vi "ProcesMTData9_2.vi"() -> ()   [LabVIEW 2018]
uses:
  <vilib>/gmath/NumericalOptimization/Nonlinear Curve Fit LM.vi
  <vilib>/gmath/statdist.llb/st_Percentiles (scalar).vi
  <vilib>/gmath/NI_Gmath.lvlib
panel:
  out "Busy with":string
  in  "test":bool
  out "Busy":bool
  in  "Fit function":u16(ring) caption="Data set" items=["Choose model ...", "WLC", "FiberWLC"]
  out "Parametersclipboard":T1(array[cluster])
  in  "Parameters":T1(array[cluster]) {"value" format="%#.2f"; "SE" format="%_2g"}
  out "Cursor positions label":string[](array[string])=["t min (s)", "t max (s)", "F min (pN)", "Fmax (pN)", "z min (um)", "z max (um)"]
  in  "Cursor positions":dbl[](array[numeric])=[0.0, 200.0, 0.0, 25.0, 0.0, 2.0]
  in  "Data set":u16(ring) caption="Trace name"
  out "F(z) graph":cluster{"Data Out":dbl[], "Data Out":dbl[]}[](graph) caption="<65535>\n\nChoose model ..."
  out "z(t) Graph":cluster{"Data Out":dbl[], "Data Out":dbl[]}[](graph)
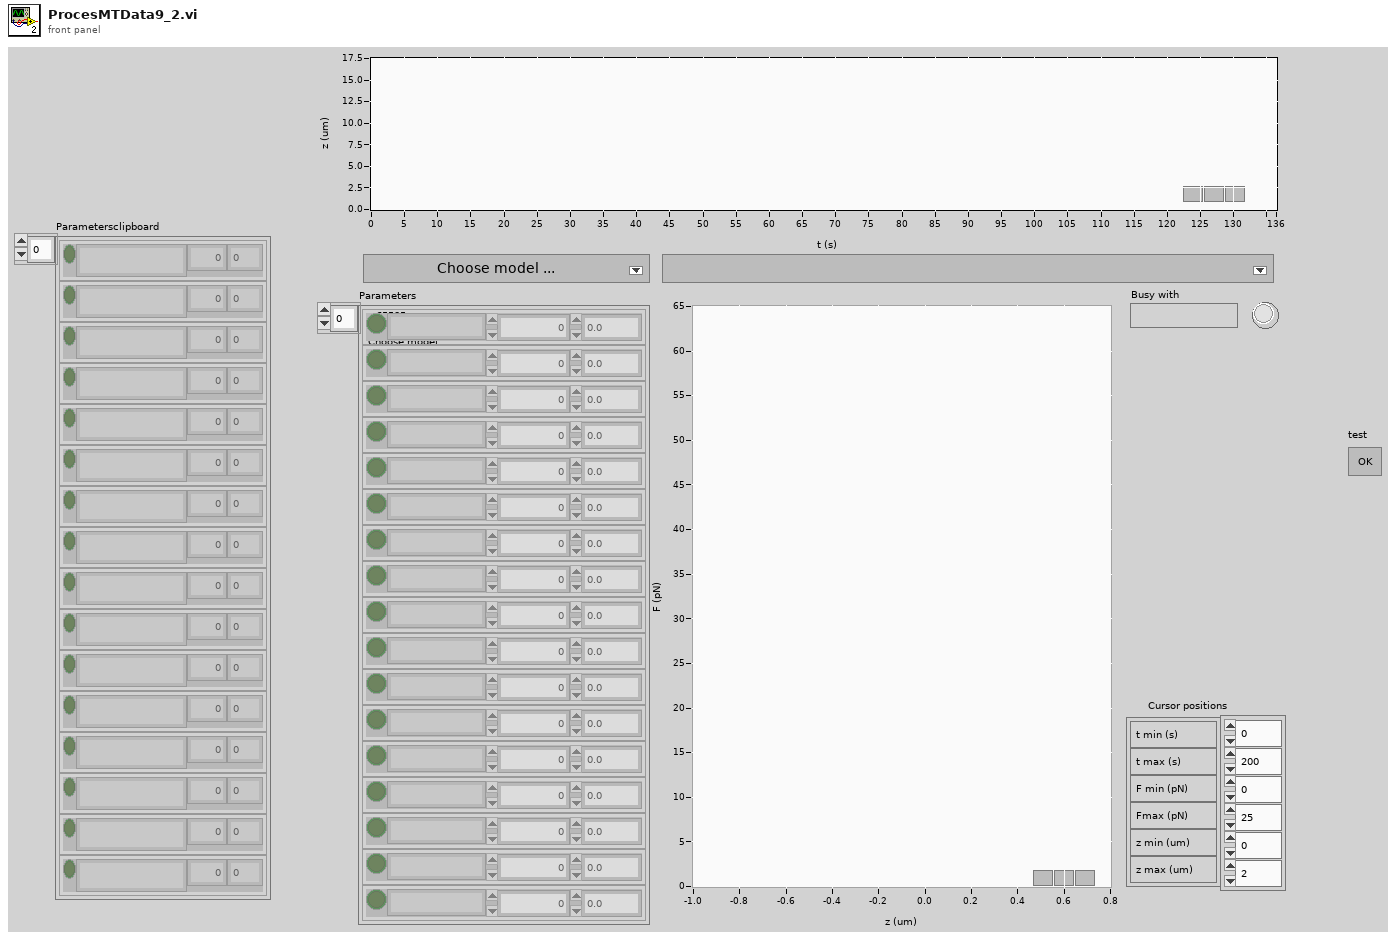
[diagram p1: front panel]
types:
  T1 = cluster{"fit":bool, "parname":string, "value":dbl, "SE":dbl}[]
  T2 = enum16{"Select all", "Select none", "Include", "Exclude"}
  T3 = enum16{"Init", "Reset", "Update var pars", "Update SE's", "Get", "Save to file", "Read from file"}
  T4 = enum16{"Read", "Write", "Get channels", "Delete channels"}
  T5 = cluster{"fit":bool, "parname":string, "value":dbl, "SE":dbl}
  T6 = cluster{bool, "ParName":string, "Value":dbl, "SE":dbl}[]
  T7 = typedef "eventvkey.ctl" = enum16{"ASCII", "Enter", "Return", "Shift", "Ctrl", "Alt", "Cmd", "Opt", "Caps", "NumLock", "Clear", "Break", "Up", "Down", "Left", "Right", "Insert", "Delete", "Home", "End", "PageUp", "PageDown", "Escape", "Help", "Pause", "ScrollLock", "F1", "F2", "F3", "F4", "F5", "F6", "F7", "F8", "F9", "F10", "F11", "F12", "F13", "F14", "F15", "F16", "F17", "F18", "F19", "F20", "F21", "F22", "F23", "F24", "Play", "VolumeUp", "VolumeDown", "Mute", "Two Byte Char"}
  T8 = enum16{"Init", "Update", "Get", "Save", "Add SE", "To text"}
  T9 = enum16{"Init", "Update", "Get", "Save", "Add SE"}
  T10 = typedef "NI_Matrix.lvlib/RealMatrix.ctl" = dbl[][]
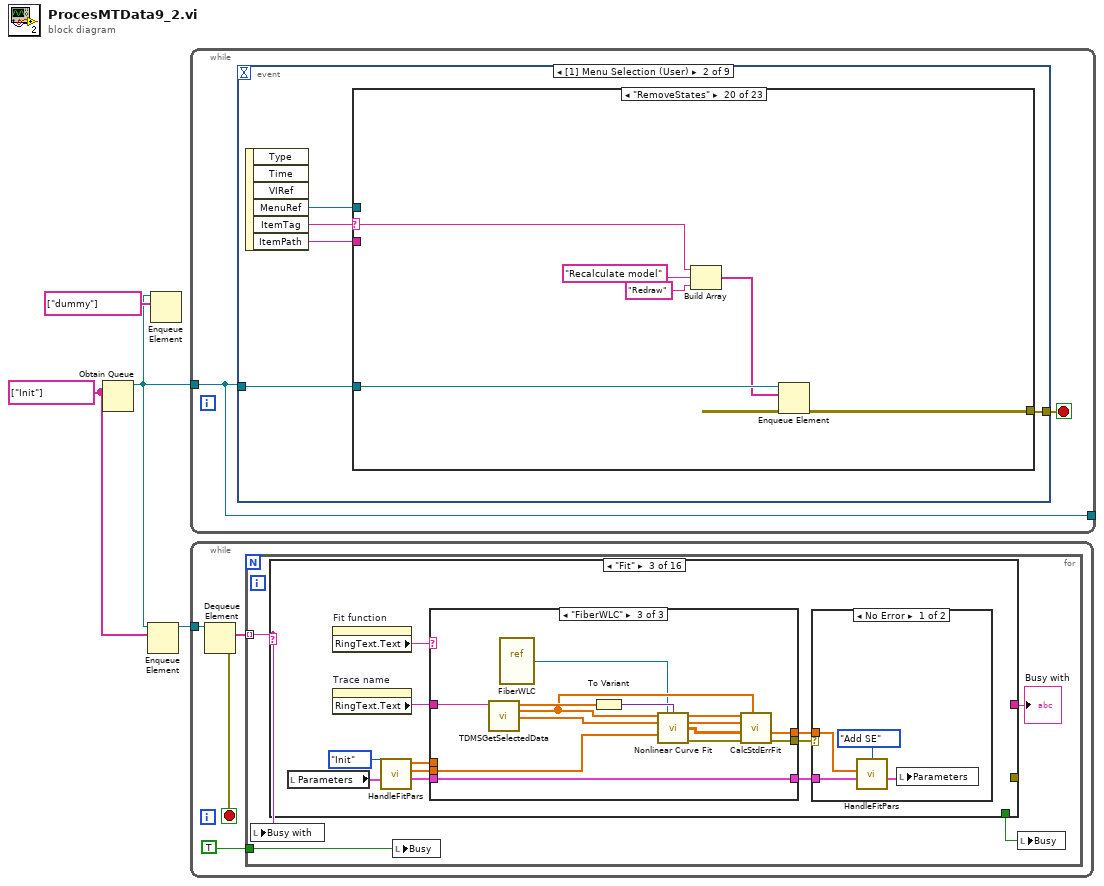
[diagram p0: block diagram]
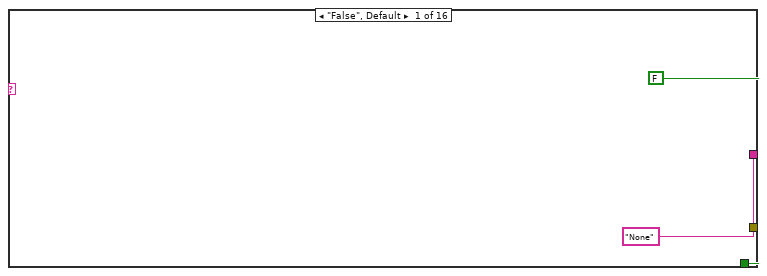
[diagram p2: hidden frame]
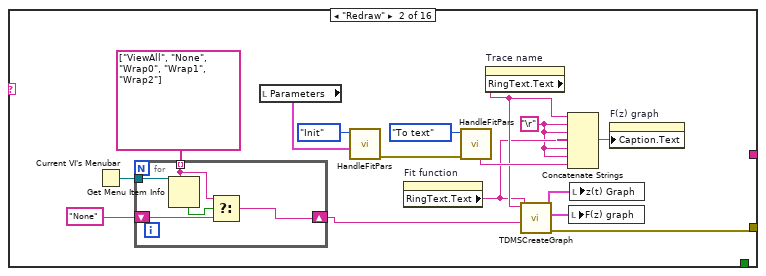
[diagram p3: hidden frame]
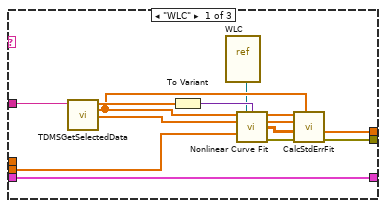
[diagram p4: hidden frame]
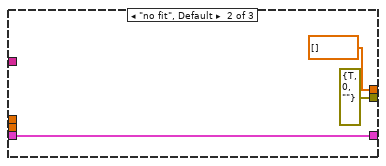
[diagram p5: hidden frame]
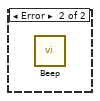
[diagram p6: hidden frame]
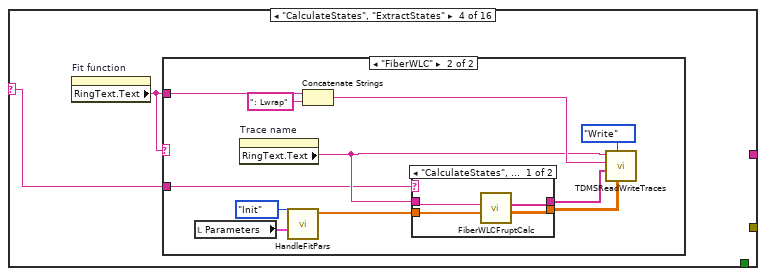
[diagram p7: hidden frame]
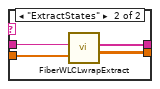
[diagram p9: hidden frame]
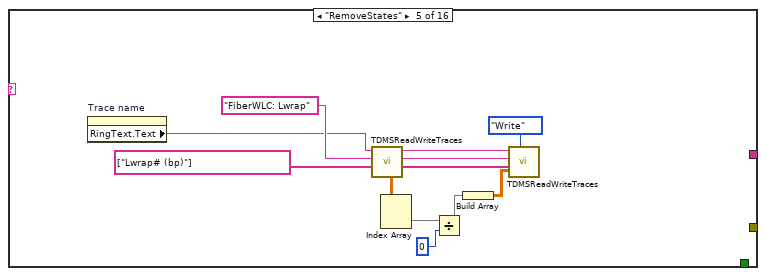
[diagram p10: hidden frame]
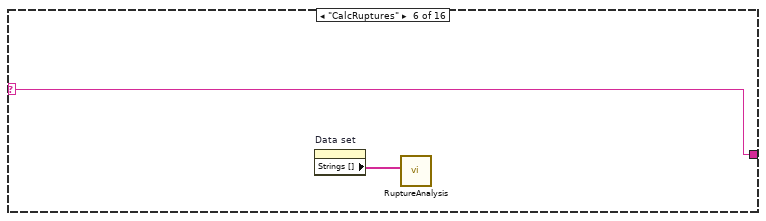
[diagram p11: hidden frame]
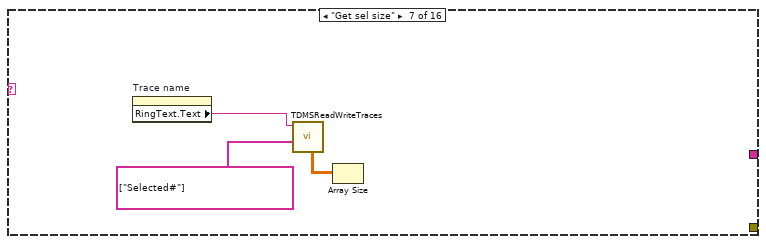
[diagram p12: hidden frame]
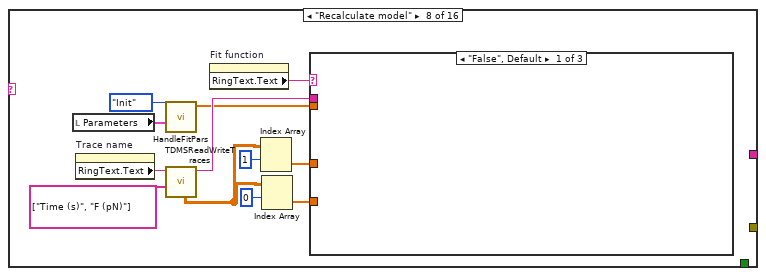
[diagram p13: hidden frame]
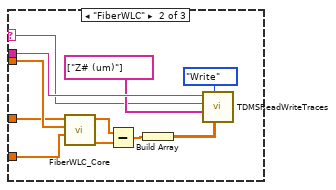
[diagram p14: hidden frame]
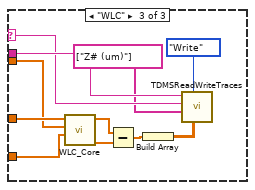
[diagram p15: hidden frame]
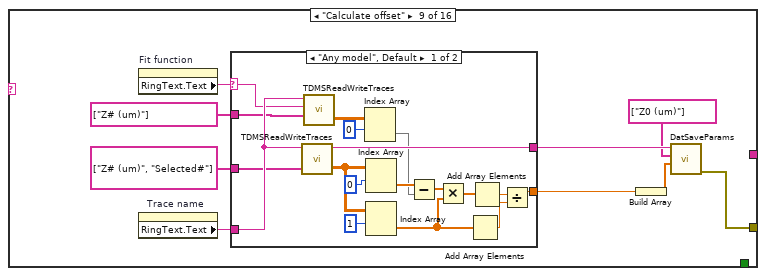
[diagram p16: hidden frame]
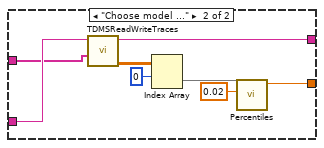
[diagram p17: hidden frame]
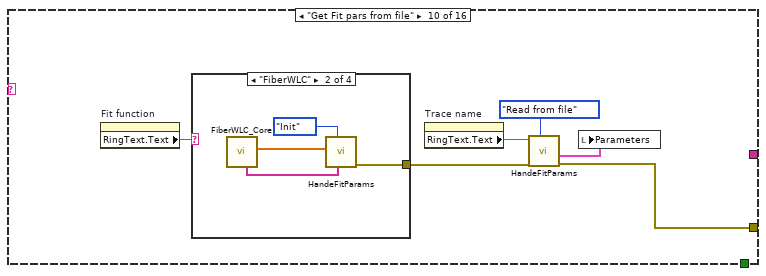
[diagram p18: hidden frame]
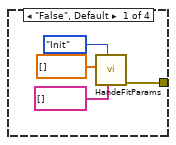
[diagram p19: hidden frame]
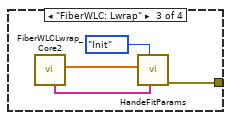
[diagram p20: hidden frame]
diagram:
  w3 = string[] ["Init"]
  n1 = Obtain Queue(element data type=w3) -> (queue out=w1:refnum<queue>)  [unwired: 4 in, 2 out]
  n2 = Enqueue Element(queue=w1, element=w3) -> (queue out=w4:refnum<queue>)  [unwired: 2 in, 2 out]
  n3 = Enqueue Element(queue=w1, element=string[] ["dummy"]) -> ()  [unwired: 2 in, 3 out]
  n4 = while {
    tunnel: w1 -> [w5]
    tunnel: [w5] -> _
    stop <- w6 stop-if-true
    n5 = event shown="[1] Menu Selection (User)" {
      selector: _ -> [_ _ _ _ _ _ _ _ _]
      dyn-events: _ -> [_ _ _ _ _ _ _ _ _]
      timeout: _ -> [_ _ _ _ _ _ _ _ _]
      tunnel: [_ w9 _ _ w399 w405 w429 _ w460] -> w6
      tunnel: w5 -> [_ w7 w376 _ w400 w407 w431 w439 w461]
      event Timeout {
        n6 = event-data() -> ()  [unwired: 1 in, 2 out]
      }
      event Menu Selection (User) {
        n7 = event-data() -> ("MenuRef"=w10:refnum<k9>, "ItemTag"=w11:string, "ItemPath"=w8:string)  [unwired: 1 in, 3 out]
        n8 = case shown="\"RemoveStates\"" w11 {
          selector: w11 -> [w17 w147 _ _ _ w180 _ _ _ _ _ _ _ _ w235 _ _ _ w307 w314 w320 w363 _]
          tunnel: w10 -> [_ w151 _ _ _ _ _ _ _ _ _ _ _ _ _ _ _ _ _ _ _ w364 _]
          tunnel: [_ _ _ _ _ _ _ _ _ _ _ errorcluster {"status"=TRUE, "code"=0, "source"=""} ("error out") _ w228 w236 w248 _ w304 w309 w315 _ _ _] -> w9
          tunnel: w8 -> [_ _ _ _ _ _ _ _ _ _ _ _ _ _ _ _ _ _ _ _ _ _ _]
          tunnel: w7 -> [w15 w145 w161 w171 w173 w176 _ _ w209 w211 _ w218 _ _ _ w250 _ w305 w310 w316 _ _ _]
          frame "Add", "All", "Constant", "Current view", "Decreasing", "Exclude", "Include", "Increasing", "Invert", "Subtract" {
            n9 = local read "Cursor positions"() -> (w16:dbl[])
            n10 = property on="Trace name" class="Ring (strict)"() -> ("RingText.Text"=w12:string)  [unwired: 2 in, 2 out]
            n11 = case shown="\"Decreasing\"" w17 {
              tunnel: w16 -> [w21 w25 w29 w38 w72 _ _ _ _ w142]
              tunnel: w12 -> [w20 w24 w28 w35 w73 w85 w99 w114 w128 w143]
              tunnel: [w18 w22 w26 w30 w62 w77 w90 w104 w119 w132] -> w13
              frame "Include", Default {
                n12 = call "TDMSSetSelection.vi"("task"=T2."Include", "min/max [t, F, z]"=w21, "tracename in"=w20) -> ("error out"=w18:errorcluster)  [unwired: 6 in, 2 out]
              }
              frame "All" {
                n13 = call "TDMSSetSelection.vi"("task"=T2."Select all", "min/max [t, F, z]"=w25, "tracename in"=w24) -> ("error out"=w22:errorcluster)  [unwired: 6 in, 2 out]
              }
              frame "Exclude" {
                n14 = call "TDMSSetSelection.vi"("task"=T2."Exclude", "min/max [t, F, z]"=w29, "tracename in"=w28) -> ("error out"=w26:errorcluster)  [unwired: 6 in, 2 out]
              }
              frame "Current view" {
                n15 = property on="F(z) graph" class="XYGraph (strict)"() -> ("YScale.Minimum"=w40:dbl, "YScale.Maximum"=w39:dbl, "XScale.Minimum"=w33:dbl, "XScale.Maximum"=w32:dbl)  [unwired: 2 in, 2 out]
                n16 = property on="z(t) Graph" class="XYGraph (strict)"() -> ("XScale.Minimum"=w42:dbl, "XScale.Maximum"=w41:dbl)  [unwired: 2 in, 2 out]
                n17 = Build Array(w42, w41, w40, w39, w33, w32) -> (w36:dbl[])
                n18 = Replace Array Subset(array=w38, new element=w36, index=0) -> (w34:dbl[])
                n19 = local write "Cursor positions"(w34) -> ()
                n20 = for {
                  tunnel: w34 -> [w43] mode=indexing
                  i -> [w44]
                  n21 = case shown="4, 5" w44 {
                    selector: w44 -> [w46 w52 w57]
                    tunnel: w43 -> [w45 w48 w53]
                    frame 0, Default {
                      n22 = property on="z(t) Graph" class="XYGraph (strict)"("Active Cursor"=w46) -> (error out=w47:errorcluster)  [unwired: 2 in, 1 out]
                      n23 = property on="z(t) Graph" class="XYGraph (strict)"(error in=w47, "Cursor.Cursor X"=w45) -> ()  [unwired: 1 in, 2 out]
                    }
                    frame 2, 3 {
                      n24 = Subtract(x=w52, y=2) -> (x-y=w49:i32)
                      n25 = property on="F(z) graph" class="XYGraph (strict)"("Active Cursor"=w49) -> (error out=w50:errorcluster)  [unwired: 2 in, 1 out]
                      n26 = property on="F(z) graph" class="XYGraph (strict)"(error in=w50, "Cursor.Cursor Y"=w48) -> ()  [unwired: 1 in, 2 out]
                    }
                    frame 4, 5 {
                      n27 = Subtract(x=w57, y=4) -> (x-y=w54:i32)
                      n28 = property on="F(z) graph" class="XYGraph (strict)"("Active Cursor"=w54) -> (error out=w55:errorcluster)  [unwired: 2 in, 1 out]
                      n29 = property on="F(z) graph" class="XYGraph (strict)"(error in=w55, "Cursor.Cursor X"=w53) -> ()  [unwired: 1 in, 2 out]
                    }
                  }
                }
                n30 = call "TDMSSetSelection.vi"("task"=T2."Include", "min/max [t, F, z]"=w34, "tracename in"=w35) -> ("error out"=w30:errorcluster)  [unwired: 6 in, 2 out]
              }
              frame "Subtract" {
                w61 = string[] ["Selected#"]
                n31 = call "TDMSReadWriteTraces.vi"("Channels in"=w61, "tracename"=w73) -> ("tracename out"=w64:string, "Data out"=w71:dbl[][])  [unwired: 4 in, 4 out]
                n32 = call "TDMSSetSelection.vi"("task"=T2."Include", "min/max [t, F, z]"=w72, "tracename in"=w64) -> ("Selected"=w69:dbl[])  [unwired: 6 in, 2 out]
                n33 = Index Array(array=w71) -> (element=w68:dbl[])  [unwired: 2 in]
                n34 = Subtract(x=w68, y=w69) -> (x-y=w67:dbl[])
                n35 = Equal?(x=1.0, y=w67) -> (x = y?=w65:bool[])
                n36 = Boolean To (0,1)(Boolean=w65) -> (0, 1=w60:i16[])
                n37 = Build Array(w60) -> (w59:i16[][])
                n38 = call "TDMSReadWriteTraces.vi"("Data in"=w59, "Task"=enum16{"Read", "Write"}."Write", "Channels in"=w61, "group name"="Selections", "tracename"=w64) -> ("error out"=w62:errorcluster)  [unwired: 1 in, 5 out]
              }
              frame "Invert" {
                w76 = string[] ["Selected#"]
                n39 = call "TDMSReadWriteTraces.vi"("Channels in"=w76, "tracename"=w85) -> ("tracename out"=w84:string, "Data out"=w79:dbl[][])  [unwired: 4 in, 4 out]
                n40 = Index Array(array=w79, index (row)=0) -> (element=w78:dbl[])  [unwired: 1 in]
                n41 = Equal To 0?(x=w78) -> (x = 0?=w83:bool[])
                n42 = Boolean To (0,1)(Boolean=w83) -> (0, 1=w82:i16[])
                n43 = Build Array(w82) -> (w75:i16[][])
                n44 = call "TDMSReadWriteTraces.vi"("Data in"=w75, "Task"=enum16{"Read", "Write"}."Write", "Channels in"=w76, "group name"="Selections", "tracename"=w84) -> ("error out"=w77:errorcluster)  [unwired: 1 in, 5 out]
              }
              frame "Decreasing" {
                n45 = call "TDMSReadWriteTraces.vi"("Channels in"=string[] ["F (pN)"], "tracename"=w99) -> ("tracename out"=w97:string, "Data out"=w98:dbl[][])  [unwired: 4 in, 4 out]
                n46 = Index Array(array=w98) -> (element=w95:dbl[])  [unwired: 2 in]
                n47 = call "Getdxdtd2dt2.vi"("Data in"=w95) -> ("first derivative"=w94:dbl[])  [unwired: 3 in, 1 out]
                n48 = Less?(x=w94, y=0.0) -> (x < y?=w93:bool[])
                n49 = Boolean To (0,1)(Boolean=w93) -> (0, 1=w92:i16[])
                n50 = Build Array(w92) -> (w88:i16[][])
                n51 = call "TDMSReadWriteTraces.vi"("Data in"=w88, "Task"=enum16{"Read", "Write"}."Write", "Channels in"=string[] ["Selected#"], "group name"="Selections", "tracename"=w97) -> ("error out"=w90:errorcluster)  [unwired: 1 in, 5 out]
              }
              frame "Constant" {
                n52 = call "TDMSReadWriteTraces.vi"("Channels in"=string[] ["Shift (mm)"], "tracename"=w114) -> ("tracename out"=w112:string, "Data out"=w113:dbl[][])  [unwired: 4 in, 4 out]
                n53 = Index Array(array=w113) -> (element=w110:dbl[])  [unwired: 2 in]
                n54 = call "Getdxdtd2dt2.vi"("Data in"=w110) -> ("first derivative"=w109:dbl[])  [unwired: 3 in, 1 out]
                n55 = Absolute Value(x=w109) -> (abs(x)=w105:dbl[])
                n56 = Less Or Equal?(x=w105, y=0.001) -> (x <= y?=w108:bool[])
                n57 = Boolean To (0,1)(Boolean=w108) -> (0, 1=w107:i16[])
                n58 = Build Array(w107) -> (w102:i16[][])
                n59 = call "TDMSReadWriteTraces.vi"("Data in"=w102, "Task"=enum16{"Read", "Write"}."Write", "Channels in"=string[] ["Selected#"], "group name"="Selections", "tracename"=w112) -> ("error out"=w104:errorcluster)  [unwired: 1 in, 5 out]
              }
              frame "Increasing" {
                n60 = call "TDMSReadWriteTraces.vi"("Channels in"=string[] ["F (pN)"], "tracename"=w128) -> ("tracename out"=w126:string, "Data out"=w127:dbl[][])  [unwired: 4 in, 4 out]
                n61 = Index Array(array=w127) -> (element=w124:dbl[])  [unwired: 2 in]
                n62 = call "Getdxdtd2dt2.vi"("Data in"=w124) -> ("first derivative"=w123:dbl[])  [unwired: 3 in, 1 out]
                n63 = Greater?(x=w123, y=0.0) -> (0:w122:bool[])
                n64 = Boolean To (0,1)(Boolean=w122) -> (0, 1=w121:i16[])
                n65 = Build Array(w121) -> (w117:i16[][])
                n66 = call "TDMSReadWriteTraces.vi"("Data in"=w117, "Task"=enum16{"Read", "Write"}."Write", "Channels in"=string[] ["Selected#"], "group name"="Selections", "tracename"=w126) -> ("error out"=w119:errorcluster)  [unwired: 1 in, 5 out]
              }
              frame "Add" {
                w130 = string[] ["Selected#"]
                n67 = call "TDMSReadWriteTraces.vi"("Channels in"=w130, "tracename"=w143) -> ("tracename out"=w137:string, "Data out"=w141:dbl[][])  [unwired: 4 in, 4 out]
                n68 = call "TDMSSetSelection.vi"("task"=T2."Include", "min/max [t, F, z]"=w142, "tracename in"=w137) -> ("Selected"=w139:dbl[])  [unwired: 6 in, 2 out]
                n69 = Index Array(array=w141) -> (element=w138:dbl[])  [unwired: 2 in]
                n70 = Add(x=w138, y=w139) -> (x+y=w133:dbl[])
                n71 = Not Equal To 0?(x=w133) -> (x != 0?=w134:bool[])
                n72 = Boolean To (0,1)(Boolean=w134) -> (0, 1=w135:i16[])
                n73 = Build Array(w135) -> (w131:i16[][])
                n74 = call "TDMSReadWriteTraces.vi"("Data in"=w131, "Task"=enum16{"Read", "Write"}."Write", "Channels in"=w130, "group name"="Selections", "tracename"=w137) -> ("error out"=w132:errorcluster)  [unwired: 1 in, 5 out]
              }
            }
            n75 = Enqueue Element(queue=w15, element=string[] ["Redraw"], error in (no error)=w13) -> ()  [unwired: 1 in, 3 out]
          }
          frame "None", "ViewAll", "Wrap0", "Wrap1", "Wrap2" {
            n76 = for {
              tunnel: w151 -> [w155]
              tunnel: string[] ["ViewAll", "None", "Wrap0", "Wrap1", "Wrap2"] -> [w154] mode=indexing
              tunnel: [w152] -> w149
              n77 = Set Menu Item Info(6:FALSE ("checked"), 7:w154, 11:w155) -> (3:w152:refnum<k9>)  [unwired: 4 in, 1 out]
            }
            n78 = Set Menu Item Info(6:TRUE ("checked"), 7:w147, 11:w149) -> (0:w144:errorcluster)  [unwired: 4 in, 1 out]
            n79 = Enqueue Element(queue=w145, element=string[] ["Redraw"], error in (no error)=w144) -> ()  [unwired: 1 in, 3 out]
          }
          frame "Close" {
            n80 = property on="Trace name" class="Ring (strict)"() -> ("Strings []"=w160:string[], "RingText.Text"=w159:string)  [unwired: 2 in, 2 out]
            n81 = Search 1D Array(1D array=w160, element=w159) -> (index of element=w166:i32)  [unwired: 1 in]
            n82 = Delete From Array(array=w160, index=w166) -> (array with subset deleted=w163:string[])  [unwired: 1 in, 1 out]
            n83 = Array Size(array=w163) -> (size(s)=w164:i32)
            n84 = case shown="1, Default" w164 {
              tunnel: [string[] ["Open file from menu"] ("Strings []") w170] -> w158
              tunnel: w163 -> [_ w170]
              frame 0 {
              }
              frame 1, Default {
              }
            }
            n85 = Decrement(x=w166) -> (x-1=w168:i32)
            n86 = In Range and Coerce(upper limit=inf, x=w168, lower limit=0.0) -> (coerced(x)=w157:dbl)  [unwired: 1 out]
            n87 = property on="Trace name" class="Ring (strict)"("Strings []"=w158, "Value"=w157) -> (error out=w156:errorcluster)  [unwired: 2 in, 1 out]
            n88 = Enqueue Element(queue=w161, element=string[] ["Redraw"], error in (no error)=w156) -> ()  [unwired: 1 in, 3 out]
          }
          frame "Offset" {
            n89 = Enqueue Element(queue=w171, element=string[] ["Calculate offset", "Get Fit pars from file", "Redraw"]) -> ()  [unwired: 2 in, 3 out]
          }
          frame "Close All" {
            n90 = Enqueue Element(queue=w173, element=string[] ["Init"]) -> ()  [unwired: 2 in, 3 out]
          }
          frame "'Paste values", "Paste both", "Paste fit", "To all datasets" {
            n91 = case shown="\"To all datasets\"" w180 {
              selector: w180 -> [w205 _]
              tunnel: [w205 "Paste both"] -> w179
              tunnel: [w204 w206] -> w178
              frame "False", Default {
                n92 = property on="Trace name" class="Ring (strict)"() -> ("RingText.Text"=w203:string)  [unwired: 2 in, 2 out]
                n93 = Build Array(w203) -> (w204:string[])
              }
              frame "To all datasets" {
                n94 = property on="Trace name" class="Ring (strict)"() -> ("Strings []"=w206:string[])  [unwired: 2 in, 2 out]
              }
            }
            n95 = for {
              tunnel: w179 -> [w185]
              tunnel: w178 -> [w182] mode=indexing
              tunnel: [w181] -> w175
              n96 = local read "Parametersclipboard"() -> (w186:T1)
              n97 = local read "Parameters"() -> (w187:T1)
              n98 = for {
                tunnel: w187 -> [w190] mode=indexing
                tunnel: w186 -> [w189] mode=indexing
                tunnel: w185 -> [w191]
                tunnel: [w188] -> w183 mode=indexing
                n99 = case shown="\"Paste values\", Default" w191 {
                  tunnel: w190 -> [w196 w202]
                  tunnel: w189 -> [w195 w201]
                  tunnel: [w192 w199] -> w188
                  frame "Paste values", Default {
                    n100 = Unbundle By Name(w195) -> ("value"=w194:dbl)
                    n101 = Bundle By Name(cluster=w196, "value"=w194, "SE"=nan) -> (w192:T5)
                  }
                  frame "Paste both" {
                    n102 = Unbundle By Name(w201) -> ("value"=w200:dbl, "fit"=w197:bool)
                    n103 = Bundle By Name(cluster=w202, "value"=w200, "fit"=w197, "SE"=nan) -> (w199:T5)
                  }
                }
              }
              n104 = call "HandeFitParams.vi"("task"=T3."Reset", "Pars in"=w183, "tracename in"=w182) -> ("error out"=w181:errorcluster)  [unwired: 5 in, 3 out]
            }
            n105 = Enqueue Element(queue=w176, element=string[] ["Save fit parameters"], error in (no error)=w175) -> ()  [unwired: 1 in, 3 out]
          }
          frame "Model" {
            n106 = call "HelpModel.vi"() -> ()  [unwired: 11 in, 1 out]
          }
          frame "Degeneracy" {
            n107 = call "HelpDegeneracy.vi"() -> ()  [unwired: 11 in, 1 out]
          }
          frame "Browse" {
            n108 = Enqueue Element(queue=w209, element=string[] ["Browse", "Redraw"]) -> ()  [unwired: 2 in, 3 out]
          }
          frame "Open" {
            n109 = Enqueue Element(queue=w211, element=string[] ["Open", "Redraw"]) -> ()  [unwired: 2 in, 3 out]
          }
          frame "ConvertDAT" {
            n110 = call "File Dialog"("pattern (all files)"="*.dat") -> ("selected path"=w214:path, "cancelled"=w213:bool)  [unwired: 11 in, 2 out]
            n111 = case shown="False" w213 {
              tunnel: w214 -> [w215 _]
              frame False {
                n112 = call "Dat2TDMS.vi"("file path"=w215) -> ()  [unwired: 10 in, 1 out]
              }
              frame True {
              }
            }
          }
          frame "Exit" {
            n113 = Release Queue(queue=w218) -> ()  [unwired: 2 in, 3 out]
            n114 = Stop(stop? (T)=TRUE) -> ()
          }
          frame "Fix all" {
            n115 = local read "Parameters"() -> (w223:T1)
            n116 = for {
              tunnel: w223 -> [w227] mode=indexing
              tunnel: [w224] -> w221 mode=indexing
              n117 = Bundle By Name(cluster=w227, "fit"=FALSE ("fix"), "SE"=nan) -> (w224:T5)
            }
            n118 = property on="Trace name" class="Ring (strict)"() -> ("RingText.Text"=w219:string)  [unwired: 2 in, 2 out]
            n119 = call "HandeFitParams.vi"("task"=T3."Reset", "Pars in"=w221, "tracename in"=w219) -> ("Pars out"=w220:T6)  [unwired: 5 in, 3 out]
            n120 = local write "Parameters"(w220) -> ()
          }
          frame "Log file" {
            n121 = property on="Data set" class="Ring (strict)"() -> ("RingText.Text"=w231:string)  [unwired: 2 in, 2 out]
            n122 = call "ChangeExtension.vi"("extension"="log", "file in"=w231) -> ("file out"=w229:string)  [unwired: 3 in, 4 out]
            n123 = Concatenate Strings("notepad.exe " ("command line"), w229) -> (w232:string)
            n124 = call <vilib>:"System Exec.vi"("command line"=w232) -> ("error out"=w228:errorcluster)  [unwired: 7 in, 3 out]
          }
          frame "LOG file", "PAR file", "TDMS file" {
            n125 = case shown="\"LOG file\", Default" w235 {
              tunnel: ["log" ("extension") "tdms" ("extension") "_par.dat" ("extension")] -> w234
              frame "LOG file", Default {
              }
              frame "TDMS file" {
              }
              frame "PAR file" {
              }
            }
            n126 = property on="Trace name" class="Ring (strict)"() -> ("RingText.Text"=w237:string)  [unwired: 2 in, 2 out]
            n127 = call "ChangeExtension.vi"("extension"=w234, "file in"=w237) -> ("Path out"=w238:path)  [unwired: 3 in, 4 out]
            n128 = Format Into String(format string="\"%s\"", w238) -> (resulting string=w240:string)  [unwired: 2 in, 1 out]
            n129 = invoke class="Process" method="Start"(reference=refnum<k24> refnum ("System.Diagnostics.Processs"), "fileName"=w240) -> (error out=w236:errorcluster)  [unwired: 2 in, 3 out]
          }
          frame "Recalculate force" {
            n130 = property on="Trace name" class="Ring (strict)"() -> ("Strings []"=w245:string[])  [unwired: 2 in, 2 out]
            n131 = call "GetUniqueFiles.vi"("Array in"=w245) -> ("Array out"=w246:string[])  [unwired: 10 in]
            n132 = call "GetForceCalibParams2.vi"() -> ("error out"=w247:errorcluster, "F1/L1/F0/F2/L2"=w252:dbl[])  [unwired: 6 in]
            n133 = case shown="No Error" w247 {
              tunnel: w252 -> [w255 _]
              tunnel: [w254 errorcluster {"status"=FALSE, "code"=0, "source"=""} ("error out")] -> w249
              tunnel: w246 -> [w253 _]
              frame No Error {
                n134 = for {
                  tunnel: w255 -> [w268]
                  tunnel: w253 -> [w265] mode=indexing
                  tunnel: [w261] -> w254
                  n135 = call "TDMSReadWriteTraces.vi"("Channels in"=string[] ["Shift (mm)"], "tracename"=w265) -> ("Group names out"=w257:string[], "tracename out"=w267:string, "Data out"=w263:dbl[][])  [unwired: 4 in, 3 out]
                  n136 = Index Array(array=w257) -> (element=w256:string)  [unwired: 1 in]
                  n137 = Index Array(array=w263) -> (element=w262:dbl[])  [unwired: 2 in]
                  n138 = call "Stepper shift to Force3.vi"("F1/L1/F0/F2/L2"=w268, "Stepper Shift"=w262) -> ("Force(pN)"=w266:dbl[])  [unwired: 4 in, 1 out]
                  n139 = Build Array(w266) -> (w260:dbl[][])
                  n140 = call "TDMSReadWriteTraces.vi"("Data in"=w260, "Task"=T4."Write", "Channels in"=string[] ["F (pN)"], "group name"=w256, "tracename"=w267) -> ("error out"=w261:errorcluster)  [unwired: 1 in, 5 out]
                }
              }
              frame Error {
              }
            }
            n141 = Enqueue Element(queue=w250, element=string[] ["Redraw"], error in (no error)=w249) -> (error out=w248:errorcluster)  [unwired: 1 in, 2 out]
          }
          frame "Autoscale" {
            n142 = local read "z(t) Graph"() -> (w296:cluster{"Data Out":dbl[], "Data Out":dbl[]}[])
            n143 = local read "F(z) graph"() -> (w290:cluster{"Data Out":dbl[], "Data Out":dbl[]}[])
            n144 = Index Array(array=w290, index=3) -> (element=w292:cluster{"Data Out":dbl[], "Data Out":dbl[]})
            n145 = Index Array(array=w296, index=3) -> (element=w294:cluster{"Data Out":dbl[], "Data Out":dbl[]})
            n146 = Unbundle(w292) -> ("Data Out"=w289:dbl[])  [unwired: 1 out]
            n147 = Unbundle(w294) -> ("Data Out"=w293:dbl[], "Data Out"=w273:dbl[])
            n148 = call-poly <vilib>:"Percentiles.vi"("p"=5.0, "x array"=w273) -> ()  [unwired: 8 in, 2 out]
            n149 = call-poly <vilib>:"Percentiles.vi"("p"=95.0, "x array"=w273) -> ()  [unwired: 8 in, 2 out]
            n150 = Array Max & Min(array=w273) -> (max value=w271:dbl, min value=w270:dbl)  [unwired: 2 out]
            n151 = Array Max & Min(array=w289) -> (max value=w287:dbl, min value=w288:dbl)  [unwired: 2 out]
            n152 = Array Max & Min(array=w293) -> (max value=w285:dbl, min value=w286:dbl)  [unwired: 2 out]
            n153 = Round Toward -Infinity(1:w286) -> (0:w277:dbl)
            n154 = Round Toward +Infinity(x=w285) -> (ceil(x): smallest int >= x=w280:dbl)
            n155 = Round Toward -Infinity(1:w270) -> (0:w276:dbl)
            n156 = Round Toward +Infinity(x=w287) -> (ceil(x): smallest int >= x=w278:dbl)
            n157 = Round Toward +Infinity(x=w271) -> (ceil(x): smallest int >= x=w279:dbl)
            n158 = Round Toward -Infinity(1:w288) -> (0:w275:dbl)
            n159 = Build Array(w277, w280) -> (w284:dbl[])
            n160 = Build Array(w276, w279) -> (w281:dbl[])
            n161 = Build Array(w275, w278) -> (w282:dbl[])
            n162 = Build Array (concatenate)(w284, w282, w281) -> (w283:dbl[])
            n163 = Index Array(array=w283) -> (element #1=w299:dbl, element #2=w300:dbl, element #3=w302:dbl, element #4=w301:dbl, element #5=w297:dbl, element #6=w298:dbl)  [unwired: 6 in]
            n164 = local write "Cursor positions"(w283) -> ()
            n165 = property on="F(z) graph" class="XYGraph (strict)"("XScale.Minimum"=w297, "XScale.Maximum"=w298, "YScale.Minimum"=w302, "YScale.Maximum"=w301) -> ()  [unwired: 2 in, 2 out]
            n166 = property on="z(t) Graph" class="XYGraph (strict)"("XScale.Maximum"=w300, "XScale.Minimum"=w299, "YScale.Maximum"=w298, "YScale.Minimum"=w297) -> ()  [unwired: 2 in, 2 out]
          }
          frame "Fit" {
            n167 = Enqueue Element(queue=w305, element=string[] ["Fit", "Write Fit pars to file", "Recalculate model", "Redraw"]) -> (error out=w304:errorcluster)  [unwired: 2 in, 2 out]
          }
          frame "CalcRuptures", "CalculateStates", "ExtractStates" {
            n168 = Build Array(w307, "Redraw") -> (w306:string[])
            n169 = Enqueue Element(queue=w310, element=w306) -> (error out=w309:errorcluster)  [unwired: 2 in, 2 out]
          }
          frame "RemoveStates" {
            n170 = Build Array(w314, "Recalculate model" ("element"), "Redraw") -> (w313:string[])
            n171 = Enqueue Element(queue=w316, element=w313) -> (error out=w315:errorcluster)  [unwired: 2 in, 2 out]
          }
          frame "BMP", "Clipboard", "EMF" {
            n172 = case shown="\"Clipboard\"" w320 {
              tunnel: [".emf" ("extension") ".bmp" ("extension") "Clipboard" ("extension")] -> w319
              tunnel: [enum32{"BMP", "EPS", "EMF", "PICT"}."EMF" ("File Type") enum32{"BMP", "EPS", "EMF", "PICT"}."BMP" ("File Type") enum32{"BMP", "EPS", "EMF", "PICT"}."BMP" ("File Type")] -> w318
              tunnel: [enum32{"File", "Clipboard"}."File" ("Target") enum32{"File", "Clipboard"}."File" ("Target") enum32{"File", "Clipboard"}."Clipboard" ("Target")] -> w317
              frame "False", Default {
              }
              frame "BMP" {
              }
              frame "Clipboard" {
              }
            }
            n173 = property on="Data set" class="Ring (strict)"() -> ("RingText.Text"=w330:string)  [unwired: 2 in, 2 out]
            n174 = call "ChangeExtension.vi"("extension"=w319, "file in"=w330) -> ("Tracenr"=w328:string, "Path out"=w329:path)  [unwired: 3 in, 3 out]
            n175 = Concatenate Strings("_" ("string"), w328, w319) -> (w326:string)
            n176 = call "ChangeExtension.vi"("extension"=w326, "Path in"=w329) -> ("Path out"=w325:path)  [unwired: 3 in, 4 out]
            n177 = call <vilib>:"Check if File or Folder Exists.vi"("path"=w325) -> ("file or folder exists?"=w323:bool, "dup path"=w324:path)  [unwired: 8 in, 1 out]
            n178 = case shown="False" w323 {
              tunnel: w324 -> [w356 w358]
              tunnel: [w356 w360] -> w322
              tunnel: [errorcluster {"status"=FALSE, "code"=0, "source"=""} ("error out") w359] -> w321
              frame False {
              }
              frame True {
                n179 = Strip Path(path=w358) -> (name=w357:string)  [unwired: 1 out]
                n180 = call "File Dialog2"("start path"=w358, "default name"=w357, "pattern (all files)"="*.bmp") -> ("selected path"=w360:path, "error out"=w359:errorcluster)  [unwired: 9 in, 2 out]
              }
            }
            n181 = case shown="No Error" w321 {
              tunnel: w322 -> [w343 _]
              tunnel: w318 -> [w341 _]
              tunnel: w317 -> [w340 _]
              frame No Error {
                w342 = TRUE ("Hide Grid")
                n182 = for {
                  N: 2 -> [_]
                  tunnel: [w352] -> w344
                  i -> [w354]
                  n183 = property on="F(z) graph" class="XYGraph (strict)"("Active Cursor"=w354, "Cursor.Visible"=FALSE ("Cursor.Watch All Plots")) -> (error out=w352:errorcluster)  [unwired: 2 in, 1 out]
                }
                n184 = invoke on="F(z) graph" class="XYGraph (strict)" method="Export Image"(error in=w344, "FileType"=w341, "Target"=w340, "Path"=w343, "HideGrid"=w342, "Overwrite"=w342) -> (error out=w345:errorcluster)  [unwired: 2 in, 7 out]
                n185 = for {
                  N: 2 -> [_]
                  tunnel: [w349] -> _
                  tunnel: w345 -> [w348]
                  i -> [w351]
                  n186 = property on="F(z) graph" class="XYGraph (strict)"(error in=w348, "Active Cursor"=w351, "Cursor.Visible"=TRUE ("Cursor.Watch All Plots")) -> (error out=w349:errorcluster)  [unwired: 1 in, 1 out]
                }
              }
              frame Error {
              }
            }
          }
          frame "Blue", "Green", "Red" {
            w368 = u32 2 ("Active Plot")
            n187 = for {
              tunnel: w364 -> [w375]
              tunnel: string[] ["Red", "Blue", "Green"] -> [w374] mode=indexing
              tunnel: [w372] -> w367
              n188 = Set Menu Item Info(6:FALSE ("checked"), 7:w374, 11:w375) -> (3:w372:refnum<k9>)  [unwired: 4 in, 1 out]
            }
            n189 = Set Menu Item Info(6:TRUE ("checked"), 7:w363, 11:w367) -> ()  [unwired: 4 in, 2 out]
            n190 = case shown="\"Green\"" w363 {
              tunnel: [u32 16860 u32 35103 u32 16711680] -> w362
              frame "Blue" {
              }
              frame "Green" {
              }
              frame "Red", Default {
              }
            }
            n191 = property on="z(t) Graph" class="XYGraph (strict)"("Active Plot"=w368, "Plot.Fill/Pt. Color"=w362) -> ()  [unwired: 2 in, 2 out]
            n192 = property on="F(z) graph" class="XYGraph (strict)"("Active Plot"=w368, "Plot.Fill/Pt. Color"=w362) -> ()  [unwired: 2 in, 2 out]
          }
          frame "other", Default {
          }
        }
      }
      event "Cursor positions": Value Change {
        n193 = event-data() -> ()  [unwired: 1 in, 5 out]
        n194 = Enqueue Element(queue=w376, element=string[] ["Update cursor positions"]) -> ()  [unwired: 2 in, 3 out]
      }
      event "z(t) Graph", "F(z) graph": Cursor Move {
        n195 = event-data() -> ()  [unwired: 1 in, 8 out]
        n196 = for {
          N: 2 -> [_]
          tunnel: [w394] -> w389 mode=indexing
          tunnel: [w393] -> w390 mode=indexing
          tunnel: [w392] -> w380 mode=indexing
          i -> [w397]
          n197 = property on="z(t) Graph" class="XYGraph (strict)"("Active Cursor"=w397) -> (error out=w396:errorcluster)  [unwired: 2 in, 1 out]
          n198 = property on="F(z) graph" class="XYGraph (strict)"("Active Cursor"=w397) -> (error out=w395:errorcluster)  [unwired: 2 in, 1 out]
          n199 = property on="F(z) graph" class="XYGraph (strict)"(error in=w395) -> ("Cursor.Cursor Y"=w394:dbl, "Cursor.Cursor X"=w392:dbl)  [unwired: 1 in, 2 out]
          n200 = property on="z(t) Graph" class="XYGraph (strict)"(error in=w396) -> ("Cursor.Cursor X"=w393:dbl)  [unwired: 1 in, 2 out]
        }
        n201 = local read "Cursor positions"() -> (w383:dbl[])
        n202 = Array Max & Min(array=w390) -> (max value=w387:dbl, min value=w388:dbl)  [unwired: 2 out]
        n203 = Array Max & Min(array=w389) -> (max value=w385:dbl, min value=w386:dbl)  [unwired: 2 out]
        n204 = Array Max & Min(array=w380) -> (max value=w379:dbl, min value=w378:dbl)  [unwired: 2 out]
        n205 = Build Array(w388, w387, w386, w385, w378, w379) -> (w382:dbl[])
        n206 = Replace Array Subset(array=w383, new element=w382, index=0) -> (w381:dbl[])
        n207 = local write "Cursor positions"(w381) -> ()
      }
      event "Data set": Value Change {
        (unwired) string[] ["Get Fit pars from file", "Recalculate model", "Redraw"] ("element")
        n208 = event-data() -> ()  [unwired: 1 in, 5 out]
        n209 = Enqueue Element(queue=w400, element=string[] ["Get Fit pars from file", "Redraw"]) -> (error out=w399:errorcluster)  [unwired: 2 in, 2 out]
      }
      event Key Down {
        n210 = event-data() -> ("VKey"=w406:T7)  [unwired: 1 in, 9 out]
        n211 = case shown="\"F12\"" w406 {
          tunnel: [errorcluster {"status"=FALSE, "code"=0, "source"=""} ("error out") w417 w423] -> w404
          tunnel: [string[] [] ("element") w416 w422] -> w403
          tunnel: string[] ["Get Fit pars from file", "Recalculate model", "Redraw"] ("element") -> [_ w416 w422]
          frame "ASCII", Default {
          }
          frame "F12" {
            n212 = property on="Data set" class="Ring (strict)"() -> ("Value"=w421:u16, "NumItems"=w420:u32)  [unwired: 2 in, 2 out]
            n213 = Increment(x=w421) -> (x+1=w419:u16)
            n214 = Decrement(x=w420) -> (x-1=w418:u32)
            n215 = Max & Min(x=w419, y=w418) -> (min(x,y)=w415:u32)  [unwired: 1 out]
            n216 = property on="Data set" class="Ring (strict)"("Val(Sgnl)"=w415) -> (error out=w417:errorcluster)  [unwired: 2 in, 1 out]
          }
          frame "F11" {
            n217 = property on="Data set" class="Ring (strict)"() -> ("Value"=w428:u16)  [unwired: 2 in, 2 out]
            n218 = To Quad Integer(1:w428) -> (0:w424:i64)
            n219 = Decrement(x=w424) -> (x-1=w427:i64)
            n220 = Max & Min(x=w427, y=u16 0) -> (max(x,y)=w425:i64)  [unwired: 1 out]
            n221 = property on="Data set" class="Ring (strict)"("Val(Sgnl)"=w425) -> (error out=w423:errorcluster)  [unwired: 2 in, 1 out]
          }
        }
        n222 = case shown="False" FALSE {
          tunnel: w407 -> [_ w412]
          tunnel: [errorcluster {"status"=FALSE, "code"=0, "source"=""} ("error out") w411] -> w405
          tunnel: w404 -> [_ w410]
          tunnel: w403 -> [_ w409]
          frame False {
          }
          frame True {
            n223 = Enqueue Element(queue=w412, element=w409, error in (no error)=w410) -> (error out=w411:errorcluster)  [unwired: 1 in, 2 out]
          }
        }
      }
      event "Fit function": Value Change {
        n224 = event-data() -> ()  [unwired: 1 in, 6 out]
        n225 = Enqueue Element(queue=w431, element=string[] ["Get Fit pars from file", "Redraw"]) -> (error out=w429:errorcluster)  [unwired: 2 in, 2 out]
      }
      event "Parameters": Value Change {
        n226 = event-data() -> ("OldVal"=w446:T1, "NewVal"=w435:T1)  [unwired: 1 in, 4 out]
        n227 = for {
          tunnel: w435 -> [w457] mode=indexing
          tunnel: w446 -> [w458] mode=indexing
          tunnel: [w449] -> w445 mode=indexing
          tunnel: [w454] -> w443 mode=indexing
          n228 = Unbundle By Name(w458) -> ("parname"=w454:string, "value"=w456:dbl, "fit"=w453:bool)
          n229 = Unbundle By Name(w457) -> ("value"=w455:dbl, "fit"=w452:bool)
          n230 = Equal?(x=w453, y=w452) -> (x = y?=w451:bool)
          n231 = Equal?(x=w456, y=w455) -> (x = y?=w450:bool)
          n232 = And(x=w450, y=w451) -> (x .and. y?=w449:bool)
        }
        n233 = Search 1D Array(1D array=w445, element=FALSE) -> (index of element=w434:i32)  [unwired: 1 in]
        n234 = Index Array(array=w435, index=w434) -> (element=w437:T5)
        n235 = Bundle By Name(cluster=w437, "SE"=nan) -> (w433:T5)
        n236 = Replace Array Subset(array=w435, new element=w433, index=w434) -> (w432:T1)
        n237 = local write "Parameters"(w432) -> ()
        n238 = Index Array(array=w443, index=w434) -> (element=w442:string)
        n239 = Search 1D Array(1D array=string[] ["Z0 (nm)", "dZ/dt (um/s)"], element=w442) -> (index of element=w440:i32)  [unwired: 1 in]
        n240 = case shown="-1" w440 {
          tunnel: [string[] ["Write Fit pars to file", "Recalculate model", "Redraw"] ("element") string[] ["Write Fit pars to file", "Redraw"] ("element")] -> w438
          frame -1 {
          }
          frame 0, Default {
          }
        }
        n241 = Enqueue Element(queue=w439, element=w438) -> ()  [unwired: 2 in, 3 out]
      }
      event "test": Value Change {
        (unwired) string[] ["Recalculate model", "Redraw"] ("element")
        (unwired) "Write Fit pars to file"
        n242 = event-data() -> ()  [unwired: 1 in, 6 out]
        n243 = Enqueue Element(queue=w461, element=string[] ["Get sel size", "Test", "Redraw"]) -> (error out=w460:errorcluster)  [unwired: 2 in, 2 out]
      }
    }
  }
  n244 = while {
    tunnel: w4 -> [w465]
    stop <- w463 stop-if-true
    n245 = Dequeue Element(queue=w465) -> (element=w464:string[], error out=w463:errorcluster)  [unwired: 2 in, 2 out]
    n246 = for {
      tunnel: [w466] -> _ mode=indexing
      tunnel: w464 -> [w466] mode=indexing
      tunnel: TRUE ("Busy") -> [w468]
      n247 = local write "Busy with"(w466) -> ()
      n248 = case shown="\"Fit\"" w466 {
        selector: w466 -> [_ _ _ w538 _ w571 _ _ _ _ _ _ w697 _ _ _]
        tunnel: [_ w485 _ _ _ _ _ _ w613 w646 _ _ w686 _ _ _] -> _
        tunnel: [FALSE ("Busy") _ _ _ _ _ _ _ _ _ _ _ _ _ _ _] -> w469
        tunnel: ["None" _ _ _ _ w571 _ _ _ _ _ _ _ _ _ _] -> w467
        frame "False", Default {
        }
        frame "Redraw" {
          w479 = "\r"
          n249 = Current VI's Menubar() -> (w478:refnum<k9>)
          n250 = for {
            tunnel: w478 -> [w492]
            tunnel: string[] ["ViewAll", "None", "Wrap0", "Wrap1", "Wrap2"] -> [w490] mode=indexing
            shift-right: [w488] -> w475
            shift-left: "None" -> [w489]
            n251 = Get Menu Item Info(7:w490, 11:w492) -> (4:w491:bool)  [unwired: 1 in, 6 out]
            n252 = Select(t=w490, s=w491, f=w489) -> (s? t:f=w488:string)
          }
          n253 = local read "Parameters"() -> (w472:T1)
          n254 = call "HandleFitPars.vi"("Parameters in"=w472, "Task"=T8."Init") -> ("error out"=w473:errorcluster)  [unwired: 3 in, 4 out]
          n255 = property on="Fit function" class="Ring (strict)"() -> ("RingText.Text"=w480:string)  [unwired: 2 in, 2 out]
          n256 = call "HandleFitPars.vi"("error in (no error)"=w473, "Task"=T8."To text") -> ("String"=w483:string)  [unwired: 3 in, 4 out]
          n257 = property on="Trace name" class="Ring (strict)"() -> ("RingText.Text"=w481:string)  [unwired: 2 in, 2 out]
          n258 = call "TDMSCreateGraph.vi"("States"=w475, "FitModel"=w480, "TraceName"=w481) -> ("error out"=w485:errorcluster, "F(z) Graph"=w487:cluster{"Data":dbl[], "Data":dbl[]}[], "z(t) Graph"=w486:cluster{"Data":dbl[], "Data":dbl[]}[])  [unwired: 6 in]
          n259 = Concatenate Strings(w481, w479, w479, w480, w479, w479, w483) -> (w482:string)
          n260 = local write "F(z) graph"(w487) -> ()
          n261 = local write "z(t) Graph"(w486) -> ()
          n262 = property on="F(z) graph" class="XYGraph (strict)"("Caption.Text"=w482) -> ()  [unwired: 2 in, 2 out]
        }
        frame "Fit" {
          n263 = local read "Parameters"() -> (w502:T1)
          n264 = property on="Fit function" class="Ring (strict)"() -> ("RingText.Text"=w496:string)  [unwired: 2 in, 2 out]
          n265 = property on="Trace name" class="Ring (strict)"() -> ("RingText.Text"=w500:string)  [unwired: 2 in, 2 out]
          n266 = call "HandleFitPars.vi"("Parameters in"=w502, "Task"=enum16{"Init", "Update", "Get"}."Init") -> ("Parameters out"=w494:T1, "Var params out"=w499:dbl[], "All params out"=w493:dbl[])  [unwired: 3 in, 2 out]
          n267 = case shown="\"FiberWLC\"" w496 {
            tunnel: w500 -> [w516 _ w533]
            tunnel: w499 -> [w512 _ w529]
            tunnel: [w510 errorcluster {"status"=TRUE, "code"=0, "source"=""} ("error out") w527] -> w498
            tunnel: [w505 dbl[] [] ("std error") w522] -> w497
            tunnel: [w503 w517 w520] -> w495
            tunnel: w494 -> [w503 w517 w520]
            tunnel: w493 -> [_ _ _]
            frame "WLC" {
              n268 = call "TDMSGetSelectedData.vi"("TraceName"=w516) -> ("F (pN)"=w513:dbl[], "Z (um)"=w506:dbl[], "Time (s)"=w514:dbl[])  [unwired: 8 in]
              n269 = To Variant(anything=w514) -> (Variant=w515:variant)
              n270 = vi-ref "WLC.vi"() -> (w504:refnum<vi>)
              n271 = call-poly <vilib>:"Nonlinear Curve Fit.vi"("Y"=w506, "f(x,a)"=w504, "data"=w515, "X"=w513, "initial parameters"=w512) -> ("best nonlinear fit"=w509:dbl[], "best fit parameters"=w508:dbl[], "covariance"=w507:T10, "error out"=w511:errorcluster)  [unwired: 5 in, 2 out]
              n272 = call "CalcStdErrFit.vi"("Y"=w506, "error in"=w511, "covariance"=w507, "Best Fit Params"=w508, "best nonlinear fit"=w509) -> ("error out"=w510:errorcluster, "std error"=w505:dbl[])  [unwired: 4 in, 1 out]
            }
            frame "no fit", Default {
            }
            frame "FiberWLC" {
              n273 = call "TDMSGetSelectedData.vi"("TraceName"=w533) -> ("F (pN)"=w530:dbl[], "Z (um)"=w523:dbl[], "Time (s)"=w531:dbl[])  [unwired: 8 in]
              n274 = vi-ref "FiberWLC.vi"() -> (w521:refnum<vi>)
              n275 = To Variant(anything=w531) -> (Variant=w532:variant)
              n276 = call-poly <vilib>:"Nonlinear Curve Fit.vi"("Y"=w523, "f(x,a)"=w521, "data"=w532, "X"=w530, "initial parameters"=w529) -> ("best nonlinear fit"=w526:dbl[], "best fit parameters"=w525:dbl[], "covariance"=w524:T10, "error out"=w528:errorcluster)  [unwired: 5 in, 2 out]
              n277 = call "CalcStdErrFit.vi"("Y"=w523, "error in"=w528, "covariance"=w524, "Best Fit Params"=w525, "best nonlinear fit"=w526) -> ("error out"=w527:errorcluster, "std error"=w522:dbl[])  [unwired: 4 in, 1 out]
            }
          }
          n278 = case shown="No Error" w498 {
            tunnel: w495 -> [w537 _]
            tunnel: w497 -> [w535 _]
            frame No Error {
              n279 = call "HandleFitPars.vi"("Parameters in"=w537, "Var params in"=w535, "Task"=T9."Add SE") -> ("Parameters out"=w536:T1)  [unwired: 2 in, 4 out]
              n280 = local write "Parameters"(w536) -> ()
            }
            frame Error {
              n281 = call <vilib>:"Beep.vi"() -> ()  [unwired: 12 in]
            }
          }
        }
        frame "CalculateStates", "ExtractStates" {
          n282 = property on="Fit function" class="Ring (strict)"() -> ("RingText.Text"=w539:string)  [unwired: 2 in, 2 out]
          n283 = case shown="\"FiberWLC\"" w539 {
            tunnel: w539 -> [_ w548]
            tunnel: w538 -> [_ w540]
            frame "False", Default {
            }
            frame "FiberWLC" {
              n284 = local read "Parameters"() -> (w550:T1)
              n285 = property on="Trace name" class="Ring (strict)"() -> ("RingText.Text"=w543:string)  [unwired: 2 in, 2 out]
              n286 = call "HandleFitPars.vi"("Parameters in"=w550, "Task"=enum16{"Init", "Update", "Get"}."Init") -> ("All params out"=w547:dbl[])  [unwired: 3 in, 4 out]
              n287 = Concatenate Strings(w548, ": Lwrap" ("string")) -> (w545:string)
              n288 = case shown="\"CalculateStates\", Default" w540 {
                tunnel: w547 -> [w553 w558]
                tunnel: w543 -> [w554 w557]
                tunnel: [w552 w556] -> w542
                tunnel: [w551 w555] -> w541
                frame "CalculateStates", Default {
                  n289 = call "FiberWLCFruptCalc.vi"("params in (all)"=w553, "tracename"=w554) -> ("Channel data"=w551:dbl[][], "Channels"=w552:string[])  [unwired: 7 in, 1 out]
                }
                frame "ExtractStates" {
                  n290 = call "FiberWLCLwrapExtract.vi"("params in (all)"=w558, "tracename"=w557) -> ("Channel data"=w555:dbl[][], "Channels"=w556:string[])  [unwired: 7 in, 1 out]
                }
              }
              n291 = call "TDMSReadWriteTraces.vi"("Data in"=w541, "Task"=enum16{"Read", "Write", "Get channels"}."Write", "Channels in"=w542, "group name"=w545, "tracename"=w543) -> ()  [unwired: 1 in, 6 out]
            }
          }
        }
        frame "RemoveStates" {
          w569 = "FiberWLC: Lwrap" ("group name")
          n292 = property on="Trace name" class="Ring (strict)"() -> ("RingText.Text"=w559:string)  [unwired: 2 in, 2 out]
          n293 = call "TDMSReadWriteTraces.vi"("Channels in"=string[] ["Lwrap# (bp)"], "group name"=w569, "tracename"=w559) -> ("Channels out"=w566:string[], "tracename out"=w565:string, "Data out"=w564:dbl[][])  [unwired: 3 in, 3 out]
          n294 = Index Array(array=w564) -> (element=w561:dbl[])  [unwired: 2 in]
          n295 = Divide(x=w561, y=0) -> (x/y=w562:dbl[])
          n296 = Build Array(w562) -> (w567:dbl[][])
          n297 = call "TDMSReadWriteTraces.vi"("Data in"=w567, "Task"=T4."Write", "Channels in"=w566, "group name"=w569, "tracename"=w565) -> ()  [unwired: 1 in, 6 out]
        }
        frame "CalcRuptures" {
          n298 = property on="Data set" class="Ring (strict)"() -> ("Strings []"=w570:string[])  [unwired: 2 in, 2 out]
          n299 = call "RuptureAnalysis.vi"("Tracenames"=w570) -> ()  [unwired: 11 in]
        }
        frame "Get sel size" {
          n300 = property on="Trace name" class="Ring (strict)"() -> ("RingText.Text"=w574:string)  [unwired: 2 in, 2 out]
          n301 = call "TDMSReadWriteTraces.vi"("Channels in"=string[] ["Selected#"], "tracename"=w574) -> ("Data out"=w572:dbl[][])  [unwired: 4 in, 5 out]
          n302 = Array Size(array=w572) -> ()  [unwired: 1 out]
        }
        frame "Recalculate model" {
          n303 = local read "Parameters"() -> (w579:T1)
          n304 = property on="Trace name" class="Ring (strict)"() -> ("RingText.Text"=w575:string)  [unwired: 2 in, 2 out]
          n305 = call "HandleFitPars.vi"("Parameters in"=w579, "Task"=enum16{"Init", "Update", "Get"}."Init") -> ("All params out"=w577:dbl[])  [unwired: 3 in, 4 out]
          n306 = call "TDMSReadWriteTraces.vi"("Channels in"=string[] ["Time (s)", "F (pN)"] ("channel name(s) in"), "tracename"=w575) -> ("tracename out"=w580:string, "Data out"=w576:dbl[][])  [unwired: 4 in, 4 out]
          n307 = property on="Fit function" class="Ring (strict)"() -> ("RingText.Text"=w585:string)  [unwired: 2 in, 2 out]
          n308 = Index Array(array=w576, index (row)=1) -> (element=w581:dbl[])  [unwired: 1 in]
          n309 = Index Array(array=w576, index (row)=0) -> (element=w582:dbl[])  [unwired: 1 in]
          n310 = case shown="\"False\", Default" w585 {
            selector: w585 -> [_ w589 w604]
            tunnel: w582 -> [_ w597 w608]
            tunnel: w581 -> [_ w587 w607]
            tunnel: w577 -> [_ w588 w606]
            tunnel: w580 -> [_ w596 w605]
            frame "False", Default {
            }
            frame "FiberWLC" {
              n311 = call "FiberWLC_Core.vi"("t (s)"=w597, "params in (all)"=w588, "F (pN)"=w587) -> ("Drift (um)"=w594:dbl[], "z (um)"=w595:dbl[])  [unwired: 5 in, 2 out]
              n312 = Subtract(x=w595, y=w594) -> (x-y=w593:dbl[])
              n313 = Build Array(w593) -> (w592:dbl[][])
              n314 = call "TDMSReadWriteTraces.vi"("Data in"=w592, "Task"=enum16{"Read", "Write"}."Write", "Channels in"=string[] ["Z# (um)"], "group name"=w589, "tracename"=w596) -> ()  [unwired: 1 in, 6 out]
            }
            frame "WLC" {
              n315 = call "WLC_Core.vi"("t (s)"=w608, "params in (all)"=w606, "F (pN)"=w607) -> ("Drift (um)"=w602:dbl[], "z (um)"=w603:dbl[])  [unwired: 5 in, 2 out]
              n316 = Subtract(x=w603, y=w602) -> (x-y=w601:dbl[])
              n317 = Build Array(w601) -> (w600:dbl[][])
              n318 = call "TDMSReadWriteTraces.vi"("Data in"=w600, "Task"=enum16{"Read", "Write"}."Write", "Channels in"=string[] ["Z# (um)"], "group name"=w604, "tracename"=w605) -> ()  [unwired: 1 in, 6 out]
            }
          }
        }
        frame "Calculate offset" {
          n319 = property on="Fit function" class="Ring (strict)"() -> ("RingText.Text"=w609:string)  [unwired: 2 in, 2 out]
          n320 = property on="Trace name" class="Ring (strict)"() -> ("RingText.Text"=w612:string)  [unwired: 2 in, 2 out]
          n321 = case shown="\"Any model\", Default" w609 {
            selector: w609 -> [w629 _]
            tunnel: [w634 w640] -> w617
            tunnel: [w618 w638] -> w614
            tunnel: w612 -> [w633 w637]
            tunnel: string[] ["Z# (um)"] ("channel name(s) in") -> [w632 _]
            tunnel: string[] ["Z# (um)", "Selected#"] ("channel name(s) in") -> [w630 w636]
            frame "Any model", Default {
              n322 = call "TDMSReadWriteTraces.vi"("Channels in"=w630, "tracename"=w633) -> ("tracename out"=w634:string, "Data out"=w627:dbl[][])  [unwired: 4 in, 4 out]
              n323 = call "TDMSReadWriteTraces.vi"("Channels in"=w632, "group name"=w629, "tracename"=w633) -> ("Data out"=w626:dbl[][])  [unwired: 3 in, 5 out]
              n324 = Index Array(array=w626, index (row)=0) -> (element=w624:dbl[])  [unwired: 1 in]
              n325 = Index Array(array=w627, index (row)=0) -> (element=w625:dbl[])  [unwired: 1 in]
              n326 = Index Array(array=w627, index (row)=1) -> (element=w621:dbl[])  [unwired: 1 in]
              n327 = Subtract(x=w625, y=w624) -> (x-y=w623:dbl[])
              n328 = Multiply(x=w623, y=w621) -> (x*y=w622:dbl[])
              n329 = Add Array Elements(numeric array=w621) -> (sum=w620:dbl)
              n330 = Add Array Elements(numeric array=w622) -> (sum=w619:dbl)
              n331 = Divide(x=w619, y=w620) -> (x/y=w618:dbl)
            }
            frame "Choose model ..." {
              n332 = call "TDMSReadWriteTraces.vi"("Channels in"=w636, "tracename"=w637) -> ("tracename out"=w640:string, "Data out"=w643:dbl[][])  [unwired: 4 in, 4 out]
              n333 = Index Array(array=w643, index (row)=0) -> (element=w639:dbl[])  [unwired: 1 in]
              n334 = call-poly <vilib>:"Percentiles.vi"("p"=0.02, "x array"=w639) -> ("percentile"=w638:dbl)  [unwired: 8 in, 1 out]
            }
          }
          n335 = Build Array(w614) -> (w615:dbl[])
          n336 = call "DatSaveParams.vi"("Values"=w615, "Names"=string[] ["Z0 (um)"], "tracename"=w617) -> ("error out"=w613:errorcluster)  [unwired: 5 in, 1 out]
        }
        frame "Get Fit pars from file" {
          n337 = property on="Fit function" class="Ring (strict)"() -> ("RingText.Text"=w645:string)  [unwired: 2 in, 2 out]
          n338 = case shown="\"FiberWLC\"" w645 {
            tunnel: [w652 w654 w660 w662] -> w644
            frame "False", Default {
              n339 = call "HandeFitParams.vi"("Par names"=string[] [], "task"=T3."Init", "Vars in"=dbl[] []) -> ("error out"=w652:errorcluster)  [unwired: 5 in, 3 out]
            }
            frame "FiberWLC" {
              n340 = call "FiberWLC_Core.vi"() -> ("default params"=w656:dbl[], "default parnames"=w655:string[])  [unwired: 8 in, 2 out]
              n341 = call "HandeFitParams.vi"("Par names"=w655, "task"=T3."Init", "Vars in"=w656) -> ("error out"=w654:errorcluster)  [unwired: 5 in, 3 out]
            }
            frame "FiberWLC: Lwrap" {
              n342 = call "FiberWLCLwrap_Core2.vi"() -> ("default params"=w659:dbl[], "default parnames"=w658:string[])  [unwired: 8 in, 2 out]
              n343 = call "HandeFitParams.vi"("Par names"=w658, "task"=T3."Init", "Vars in"=w659) -> ("error out"=w660:errorcluster)  [unwired: 5 in, 3 out]
            }
            frame "WLC" {
              n344 = call "WLC_Core.vi"() -> ("default params"=w664:dbl[], "default parnames"=w663:string[])  [unwired: 8 in, 2 out]
              n345 = call "HandeFitParams.vi"("Par names"=w663, "task"=T3."Init", "Vars in"=w664) -> ("error out"=w662:errorcluster)  [unwired: 5 in, 3 out]
            }
          }
          n346 = property on="Trace name" class="Ring (strict)"() -> ("RingText.Text"=w648:string)  [unwired: 2 in, 2 out]
          n347 = call "HandeFitParams.vi"("task"=T3."Read from file", "error in (no error)"=w644, "tracename in"=w648) -> ("error out"=w646:errorcluster, "Pars out"=w649:T6)  [unwired: 5 in, 2 out]
          n348 = local write "Parameters"(w649) -> ()
        }
        frame "Write Fit pars to file" {
          n349 = property on="Trace name" class="Ring (strict)"() -> ("RingText.Text"=w668:string)  [unwired: 2 in, 2 out]
          n350 = local read "Parameters"() -> (w673:T1)
          n351 = for {
            tunnel: w673 -> [w679] mode=indexing
            tunnel: [w677] -> w670 mode=indexing
            tunnel: [w678] -> w672 mode=indexing
            tunnel: [w675] -> w669 mode=indexing
            tunnel: [w674] -> w671 mode=indexing
            n352 = Unbundle By Name(w679) -> ("parname"=w677:string, "value"=w678:dbl, "SE"=w674:dbl)
            n353 = Concatenate Strings("SE: " ("string"), w677) -> (w675:string)
          }
          n354 = Build Array (concatenate)(w670, w669) -> (w667:string[])
          n355 = Build Array (concatenate)(w672, w671) -> (w666:dbl[])
          n356 = call "DatSaveParams.vi"("Values"=w666, "Names"=w667, "tracename"=w668) -> ()  [unwired: 5 in, 2 out]
        }
        frame "Test" {
          n357 = property on="Trace name" class="Ring (strict)"() -> ("RingText.Text"=w684:string)  [unwired: 2 in, 2 out]
          n358 = call "ChangeExtension.vi"("extension"="_copy.tdms", "file in"=w684) -> ("Path out"=w680:path)  [unwired: 3 in, 4 out]
          n359 = call "ChangeExtension.vi"("extension"="tdms", "file in"=w684) -> ("Path out"=w681:path)  [unwired: 3 in, 4 out]
          n360 = Copy(9:TRUE ("overwrite (F)"), 10:w681, 11:w680) -> ()  [unwired: 2 in, 3 out]
        }
        frame "Browse", "Open" {
          n361 = case shown="\"Browse\", Default" w697 {
            tunnel: [w699 w700] -> w698
            frame "Browse", Default {
              n362 = call "BrowseTDMSFile.vi"() -> ("Selected traces"=w699:string[])  [unwired: 10 in, 1 out]
            }
            frame "Open" {
              n363 = call "DatGetTraceNrs.vi"() -> ("Selected Traces"=w700:string[])  [unwired: 7 in, 4 out]
            }
          }
          n364 = property on="Trace name" class="Ring (strict)"() -> ("Strings []"=w693:string[])  [unwired: 2 in, 2 out]
          n365 = Search 1D Array(1D array=w693, element="Open file from menu") -> (index of element=w695:i32)  [unwired: 1 in]
          n366 = Delete From Array(array=w693, length=1, index=w695) -> (array with subset deleted=w692:string[])  [unwired: 1 out]
          n367 = for {
            tunnel: w698 -> [w701] mode=indexing
            shift-right: [w702] -> w691
            shift-left: w692 -> [w703]
            tunnel: [w701] -> w689 mode=indexing
            n368 = Search 1D Array(1D array=w703, element=w701) -> (index of element=w704:i32)  [unwired: 1 in]
            n369 = case shown="0, Default" w704 {
              tunnel: w703 -> [w705 w708]
              tunnel: w701 -> [_ w707]
              tunnel: [w705 w706] -> w702
              frame 0, Default {
              }
              frame -1 {
                n370 = Build Array (concatenate)(w708, w707) -> (w706:string[])
              }
            }
          }
          n371 = Index Array(array=w689) -> (element=w688:string)  [unwired: 1 in]
          n372 = Sort 1D Array(array=w691) -> (sorted array=w690:string[])
          n373 = Search 1D Array(1D array=w690, element=w688) -> (index of element=w687:i32)  [unwired: 1 in]
          n374 = property on="Trace name" class="Ring (strict)"("Strings []"=w690, "Value"=w687) -> (error out=w686:errorcluster)  [unwired: 2 in, 1 out]
        }
        frame "Update cursor positions" {
          n375 = Reshape Array("Cursor positions", 3 ("dimension size"), 2 ("dimension size")) -> (w712:dbl[][])
          n376 = for {
            tunnel: w712 -> [w721] mode=indexing
            shift-right: [w716] -> w714
            shift-left: dbl[] [] -> [w717]
            i -> [w719]
            n377 = Array Max & Min(array=w721) -> (max value=w720:dbl, min value=w718:dbl)  [unwired: 2 out]
            n378 = Build Array(w718, w720) -> (w715:dbl[])
            n379 = Build Array (concatenate)(w717, w715) -> (w716:dbl[])
            n380 = case shown="0, Default" w719 {
              tunnel: w715 -> [w722 w726 w730]
              frame 0, Default {
                # "time"
                n381 = for {
                  tunnel: w722 -> [w723] mode=indexing
                  i -> [w724]
                  n382 = property on="z(t) Graph" class="XYGraph (strict)"("Active Cursor"=w724) -> (error out=w725:errorcluster)  [unwired: 2 in, 1 out]
                  n383 = property on="z(t) Graph" class="XYGraph (strict)"(error in=w725, "Cursor.Cursor X"=w723) -> ()  [unwired: 1 in, 2 out]
                }
              }
              frame 1 {
                # "Force"
                n384 = for {
                  tunnel: w726 -> [w727] mode=indexing
                  i -> [w728]
                  n385 = property on="F(z) graph" class="XYGraph (strict)"("Active Cursor"=w728) -> (error out=w729:errorcluster)  [unwired: 2 in, 1 out]
                  n386 = property on="F(z) graph" class="XYGraph (strict)"(error in=w729, "Cursor.Cursor Y"=w727) -> ()  [unwired: 1 in, 2 out]
                }
              }
              frame 2 {
                # "z"
                n387 = for {
                  tunnel: w730 -> [w731] mode=indexing
                  i -> [w732]
                  n388 = property on="F(z) graph" class="XYGraph (strict)"("Active Cursor"=w732) -> (error out=w733:errorcluster)  [unwired: 2 in, 1 out]
                  n389 = property on="F(z) graph" class="XYGraph (strict)"(error in=w733, "Cursor.Cursor X"=w731) -> ()  [unwired: 1 in, 2 out]
                }
              }
            }
          }
          n390 = local write "Cursor positions"(w714) -> ()
        }
        frame "Init" {
          w740 = 3 ("y")
          w737 = cluster{"t (s)":dbl[], "z (um) all":dbl[]}[] [{"t (s)"=[0.0], "z (um) all"=[0.0]}, {"t (s)"=[0.0], "z (um) all"=[0.0]}, {"t (s)"=[0.0], "z (um) all"=[0.0]}, {"t (s)"=[0.0], "z (um) all"=[0.0]}, {"t (s)"=[0.0], "z (um) all"=[0.0]}, {"t (s)"=[0.0], "z (um) all"=[0.0]}, {"t (s)"=[0.0], "z (um) all"=[0.0]}, {"t (s)"=[0.0], "z (um) all"=[0.0]}, {"t (s)"=[0.0], "z (um) all"=[0.0]}, {"t (s)"=[0.0], "z (um) all"=[0.0]}, {"t (s)"=[0.0], "z (um) all"=[0.0]}, {"t (s)"=[0.0], "z (um) all"=[0.0]}, {"t (s)"=[0.0], "z (um) all"=[0.0]}, {"t (s)"=[0.0], "z (um) all"=[0.0]}, {"t (s)"=[0.0], "z (um) all"=[0.0]}, {"t (s)"=[0.0], "z (um) all"=[0.0]}, {"t (s)"=[0.0], "z (um) all"=[0.0]}, {"t (s)"=[0.0], "z (um) all"=[0.0]}, {"t (s)"=[0.0], "z (um) all"=[0.0]}, {"t (s)"=[0.0], "z (um) all"=[0.0]}, {"t (s)"=[0.0], "z (um) all"=[0.0]}, {"t (s)"=[0.0], "z (um) all"=[0.0]}, {"t (s)"=[0.0], "z (um) all"=[0.0]}, {"t (s)"=[0.0], "z (um) all"=[0.0]}, {"t (s)"=[0.0], "z (um) all"=[0.0]}, {"t (s)"=[0.0], "z (um) all"=[0.0]}, {"t (s)"=[0.0], "z (um) all"=[0.0]}, {"t (s)"=[0.0], "z (um) all"=[0.0]}, {"t (s)"=[0.0], "z (um) all"=[0.0]}, {"t (s)"=[0.0], "z (um) all"=[0.0]}, {"t (s)"=[0.0], "z (um) all"=[0.0]}, {"t (s)"=[0.0], "z (um) all"=[0.0]}, {"t (s)"=[0.0], "z (um) all"=[0.0]}, {"t (s)"=[0.0], "z (um) all"=[0.0]}, {"t (s)"=[0.0], "z (um) all"=[0.0]}, {"t (s)"=[0.0], "z (um) all"=[0.0]}, {"t (s)"=[0.0], "z (um) all"=[0.0]}, {"t (s)"=[0.0], "z (um) all"=[0.0]}, {"t (s)"=[0.0], "z (um) all"=[0.0]}, {"t (s)"=[0.0], "z (um) all"=[0.0]}, {"t (s)"=[0.0], "z (um) all"=[0.0]}, {"t (s)"=[0.0], "z (um) all"=[0.0]}, {"t (s)"=[0.0], "z (um) all"=[0.0]}, {"t (s)"=[0.0], "z (um) all"=[0.0]}, {"t (s)"=[0.0], "z (um) all"=[0.0]}, {"t (s)"=[0.0], "z (um) all"=[0.0]}, {"t (s)"=[0.0], "z (um) all"=[0.0]}, {"t (s)"=[0.0], "z (um) all"=[0.0]}, {"t (s)"=[0.0], "z (um) all"=[0.0]}, {"t (s)"=[0.0], "z (um) all"=[0.0]}, {"t (s)"=[0.0], "z (um) all"=[0.0]}, {"t (s)"=[0.0], "z (um) all"=[0.0]}, {"t (s)"=[0.0], "z (um) all"=[0.0]}, {"t (s)"=[0.0], "z (um) all"=[0.0]}, {"t (s)"=[0.0], "z (um) all"=[0.0]}, {"t (s)"=[0.0], "z (um) all"=[0.0]}, {"t (s)"=[0.0], "z (um) all"=[0.0]}, {"t (s)"=[0.0], "z (um) all"=[0.0]}, {"t (s)"=[0.0], "z (um) all"=[0.0]}, {"t (s)"=[0.0], "z (um) all"=[0.0]}, {"t (s)"=[0.0], "z (um) all"=[0.0]}, {"t (s)"=[0.0], "z (um) all"=[0.0]}, {"t (s)"=[0.0], "z (um) all"=[0.0]}, {"t (s)"=[0.0], "z (um) all"=[0.0]}, {"t (s)"=[0.0], "z (um) all"=[0.0]}, {"t (s)"=[0.0], "z (um) all"=[0.0]}, {"t (s)"=[0.0], "z (um) all"=[0.0]}, {"t (s)"=[0.0], "z (um) all"=[0.0]}, {"t (s)"=[0.0], "z (um) all"=[0.0]}, {"t (s)"=[0.0], "z (um) all"=[0.0]}, {"t (s)"=[0.0], "z (um) all"=[0.0]}, {"t (s)"=[0.0], "z (um) all"=[0.0]}, {"t (s)"=[0.0], "z (um) all"=[0.0]}, {"t (s)"=[0.0], "z (um) all"=[0.0]}, {"t (s)"=[0.0], "z (um) all"=[0.0]}, {"t (s)"=[0.0], "z (um) all"=[0.0]}, {"t (s)"=[0.0], "z (um) all"=[0.0]}, {"t (s)"=[0.0], "z (um) all"=[0.0]}, {"t (s)"=[0.0], "z (um) all"=[0.0]}, {"t (s)"=[0.0], "z (um) all"=[0.0]}, {"t (s)"=[0.0], "z (um) all"=[0.0]}, {"t (s)"=[0.0], "z (um) all"=[0.0]}, {"t (s)"=[0.0], "z (um) all"=[0.0]}, {"t (s)"=[0.0], "z (um) all"=[0.0]}, {"t (s)"=[0.0], "z (um) all"=[0.0]}, {"t (s)"=[0.0], "z (um) all"=[0.0]}, {"t (s)"=[0.0], "z (um) all"=[0.0]}, {"t (s)"=[0.0], "z (um) all"=[0.0]}, {"t (s)"=[0.0], "z (um) all"=[0.0]}, {"t (s)"=[0.0], "z (um) all"=[0.0]}, {"t (s)"=[0.0], "z (um) all"=[0.0]}, {"t (s)"=[0.0], "z (um) all"=[0.0]}, {"t (s)"=[0.0], "z (um) all"=[0.0]}, {"t (s)"=[0.0], "z (um) all"=[0.0]}, {"t (s)"=[0.0], "z (um) all"=[0.0]}, {"t (s)"=[0.0], "z (um) all"=[0.0]}, {"t (s)"=[0.0], "z (um) all"=[0.0]}, {"t (s)"=[0.0], "z (um) all"=[0.0]}, {"t (s)"=[0.0], "z (um) all"=[0.0]}, {"t (s)"=[0.0], "z (um) all"=[0.0]}]  # Empty plots
          w734 = u16 0 items=["Choose model ...", "FiberWLC", "FiberWLC : Lfree"] ("Fit function")
          # "Initialize  controls/indicators"
          n391 = property on="Fit function" class="Ring (strict)"("Value"=w734, "Strings []"=string[] ["Choose model ...", "WLC", "FiberWLC"]) -> ()  [unwired: 2 in, 2 out]
          n392 = local write "F(z) graph"(w737) -> ()
          n393 = local write "z(t) Graph"(w737) -> ()
          n394 = Array Size(array=w737) -> (size(s)=w738:i32)
          n395 = Subtract(x=w738, y=w740) -> (x-y=w739:i32)
          n396 = for {
            N: w739 -> [_]
            tunnel: w740 -> [w747]
            i -> [w748]
            w744 = u8 2 ("Plot.Line Style")
            w745 = u32 0 ("Plot.Plot Color")
            n397 = Add(x=w747, y=w748) -> (x+y=w746:i32)
            n398 = property on="z(t) Graph" class="XYGraph (strict)"("Active Plot"=w746, "Plot.Plot Color"=w745, "Plot.Line Style"=w744) -> ()  [unwired: 2 in, 2 out]
            n399 = property on="F(z) graph" class="XYGraph (strict)"("Active Plot"=w746, "Plot.Plot Color"=w745, "Plot.Line Style"=w744) -> ()  [unwired: 2 in, 2 out]
          }
          n400 = property on="Data set" class="Ring (strict)"("Strings []"=string[] ["Open file from menu"], "Value"=0) -> ()  [unwired: 2 in, 2 out]
          n401 = local write "Cursor positions"(dbl[] [0.0, 200.0, 0.0, 25.0, 0.0, 2.0] ("Cursor positions {Time, Force, Extension}")) -> ()
          n402 = local write "Parameters"(T1 [] ("Fit settings")) -> ()
        }
        frame "Dummy" {
          # "Container for all controls/indicators"
        }
      }
      "Busy with" <- w467
      n403 = local write "Busy"(w468) -> ()
      n404 = local write "Busy"(w469) -> ()
    }
  }
